vi "FlatToRichnixnet_grpc_DbDeployResponse.vi"(5 "OutputClusterType":T1, 11 "InputCluster":T2) -> (3 "OutputCluster":T1)   [LabVIEW 2025, in "grpc-xnet_client.lvlib"]
uses:
  grpc-xnet_client.lvlib
  nixnet_grpc_DbDeployResponse_Flat.ctl
  nixnet_grpc_DbDeployResponse.ctl
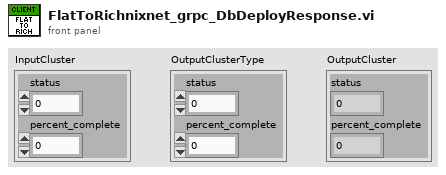
[diagram p1: front panel]
types:
  T1 = typedef "grpc-xnet_client.lvlib/nixnet_grpc_DbDeployResponse.ctl" = cluster{"status":i32, "percent_complete":u32}
  T2 = typedef "grpc-xnet_client.lvlib/nixnet_grpc_DbDeployResponse_Flat.ctl" = cluster{"status":i32, "percent_complete":u32}
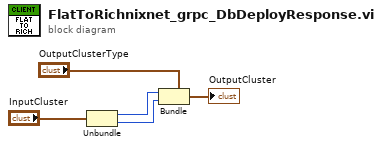
[diagram p0: block diagram]
diagram:
  n1 = Unbundle "Unbundle"("InputCluster") -> ("status"=w2:i32, "percent_complete"=w1:u32)
  n2 = Bundle "Bundle"(cluster="OutputClusterType", "status"=w2, "percent_complete"=w1) -> (→"OutputCluster":T1)
